vi "OEE_SCREEN_1_get_last_operator.vi"(8 "error_in":errorcluster, 10 "current_time_in":string, 11 "reference_name_in":string) -> (0 "error_out":errorcluster, 2 "current_time_out":string, 3 "reference_name_out":string)   [LabVIEW 2019]
uses:
  FGV/SQL_connection/FGV_OEE_SQL_connection.ctl
  FGV/SQL_raw_data/FGV_OEE_SQL_raw_data.ctl
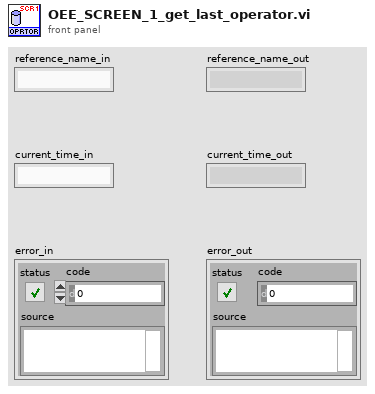
[diagram p1: front panel]
types:
  T1 = typedef "FGV_OEE_SQL_raw_data.ctl" = enum16{"initialize", "set_reference_name", "set_timestamp", "set_OK_NOK_count", "set_config_info", "set_pace", "set_availability", "set_hourly_ok_count", "set_targets", "get_all_info"}
  T2 = typedef "FGV_OEE_SQL_connection.ctl" = enum16{"initialize", "connect", "read_tables", "read_columns", "SELECT", "INSERT", "UPDATE", "DELETE", "EXEC + headers", "EXEC", "TRANSACTION", "connection_active?", "disconnect"}
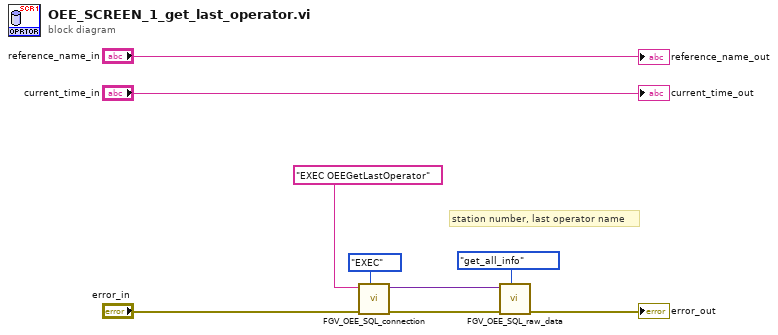
[diagram p0: block diagram]
diagram:
  # "station number, last operator name"
  n1 = call "FGV_OEE_SQL_connection.vi"("options"=FGV_OEE_SQL_connection."EXEC", "error_in"="error_in", "SQL_statement"="EXEC OEEGetLastOperator" ("format string")) -> ("error_out"=w5:errorcluster, "SQL_result"=w2:variant)  [unwired: 4 in, 3 out]
  n2 = call "FGV_OEE_SQL_raw_data.vi"("options"=FGV_OEE_SQL_raw_data."get_all_info", "error_in"=w5, "input"=w2) -> ("error_out"=→"error_out":errorcluster)  [unwired: 7 in, 1 out]
  "reference_name_out" <- "reference_name_in"
  "current_time_out" <- "current_time_in"
